vi "Send Panel Close.vi"(6 "Name (use VI name)":string, 8 "Discarded?":bool, 9 "Time":u32, 10 "VI Refnum":refnum<vi>, 11 "Message Enqueuer in":refnum<class "Message Enqueuer.lvclass">) -> (0 "error out":errorcluster)   [LabVIEW 2015, in "ActorAutoRegistration.lvlib" / "PanelCloseMsg.lvclass"]
uses:
  PanelCloseMsg.lvclass
  <vilib>/ActorFramework/Message Enqueuer/Message Enqueuer.lvclass
  PanelCloseMsg.lvclass/PanelCloseMsg.ctl
  EventDataMessage/EventDataMessage.lvclass
panel:
  in  "error in (no error)":errorcluster
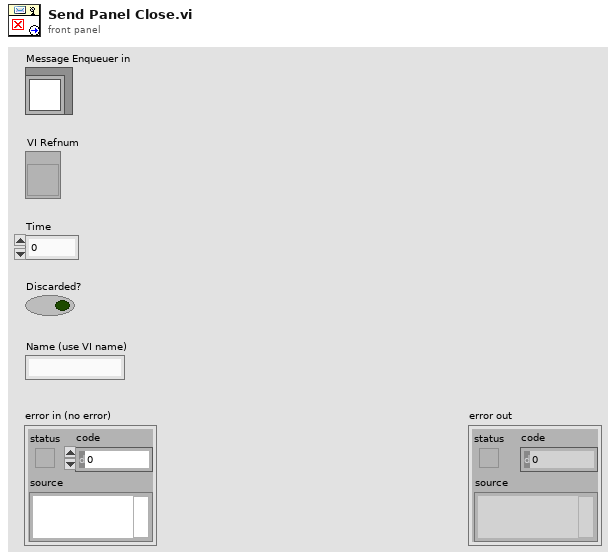
[diagram p1: front panel]
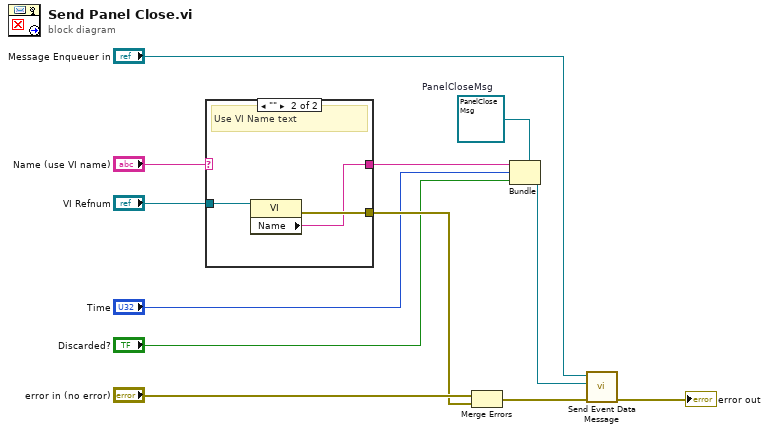
[diagram p0: block diagram]
diagram:
  w9 = refnum<class "PanelCloseMsg.lvclass"> refnum  # PanelCloseMsg
  n1 = case shown="\"\"" "Name (use VI name)" {
    selector: "Name (use VI name)" -> [w13 _]
    tunnel: [w13 w14] -> w12
    tunnel: "VI Refnum" -> [_ w16]
    tunnel: [_ w15] -> w6
    frame Default {
      # "Use string provided"
    }
    frame "" {
      # "Use VI Name text"
      n2 = property class="VI"(reference=w16) -> (error out=w15:errorcluster, "Name"=w14:string)  [unwired: 1 in, 1 out]
    }
  }
  n3 = Merge Errors("error in (no error)", w6) -> (w7:errorcluster)
  n4 = Bundle(cluster=w9, w12, "Time", "Discarded?") -> (w4:refnum<class "PanelCloseMsg.lvclass">)
  n5 = call "Send Event Data Message.vi"("error in (no error)"=w7, "EventDataMessage in"=w4, "Message Enqueuer in"="Message Enqueuer in") -> ("error out"=→"error out":errorcluster)  [unwired: 8 in]
